vi "parser.vi"(11 "input string":string) -> ()   [LabVIEW 2014]
panel:
  out "element":i32
  out "errorstate":string
  out "error":bool
  in  "Listbox":i32(listbox)
  out "Enum":enum16{"%g", "bias", "current", "frame"}(ring)
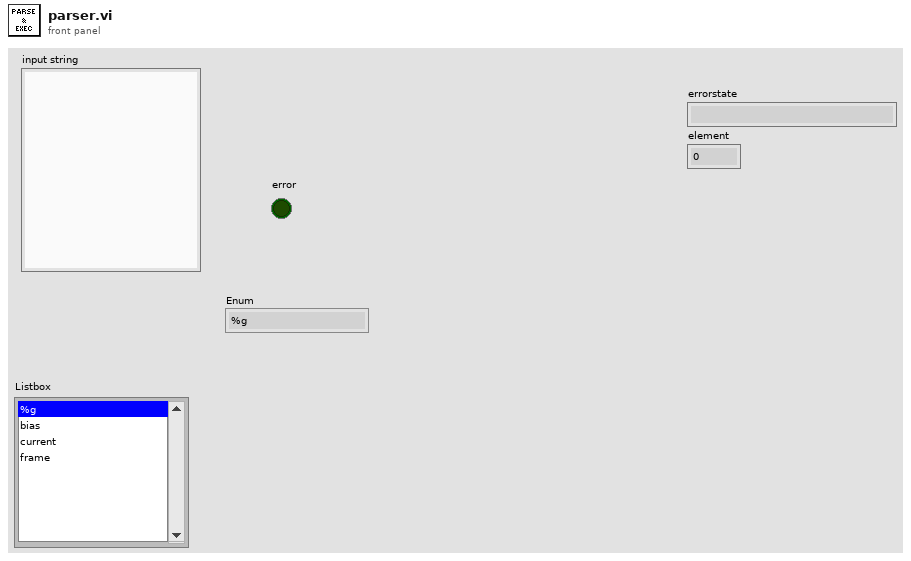
[diagram p1: front panel]
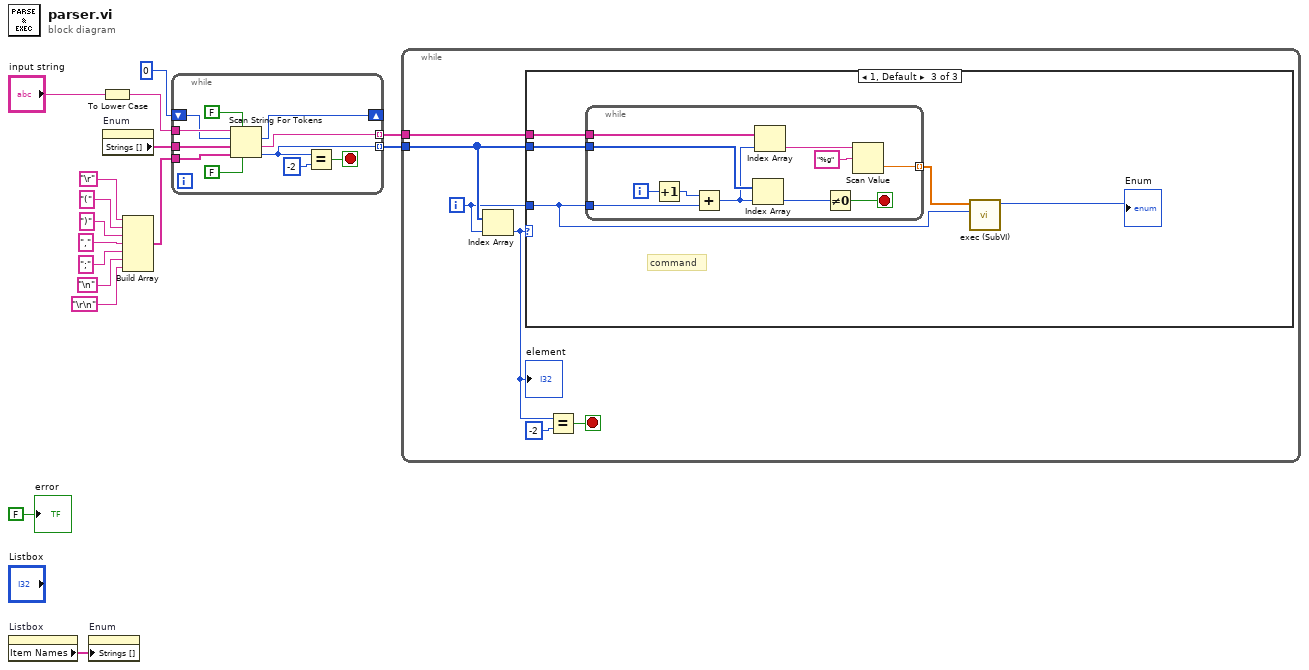
[diagram p0: block diagram]
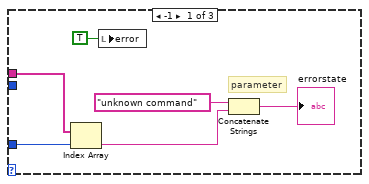
[diagram p2: hidden frame]
diagram:
  n1 = property on="Listbox" class="LstBox (strict)"() -> ("Item Names"=w4:string[])  [unwired: 2 in, 2 out]
  n2 = property on="Enum" class="Enum (strict)"("Strings []"=w4) -> ()  [unwired: 2 in, 2 out]
  n3 = To Lower Case(string="input string") -> (all lower case string=w10:string)
  n4 = property on="Enum" class="Enum (strict)"() -> ("Strings []"=w5:string[])  [unwired: 2 in, 2 out]
  n5 = Build Array("\r", "(" ("element"), ")" ("element"), "," ("element"), ";" ("element"), "\n", "\r\n") -> (w15:string[])
  n6 = while {
    tunnel: w15 -> [w27]
    tunnel: [w25] -> w6 mode=indexing
    tunnel: w5 -> [w18]
    tunnel: w10 -> [w24]
    shift-right: [w20] -> _
    shift-left: 0 ("y") -> [w21]
    tunnel: [w19] -> w7 mode=indexing
    stop <- w23 stop-if-true
    n7 = Scan String For Tokens(4:FALSE ("use cached delim/oper data? (F)"), 5:FALSE ("allow empty tokens? (F)"), 6:w27, 7:w18, 8:w21, 9:w24) -> (0:w19:i32, 1:w25:string, 2:w20:i32)  [unwired: 1 out]
    n8 = Equal?(x=w19, y=-2) -> (x = y?=w23:bool)
  }
  n9 = while {
    tunnel: w7 -> [w31]
    tunnel: w6 -> [w29]
    i -> [w30]
    stop <- w32 stop-if-true
    n10 = Index Array(array=w31, index=w30) -> (element=w28:i32)
    "element" <- w28
    n11 = case shown="1, Default" w28 {
      tunnel: w31 -> [_ _ w44]
      tunnel: w30 -> [w37 _ w42]
      tunnel: w29 -> [w38 _ w43]
      frame -1 {
        # "parameter"
        n12 = Index Array(array=w38, index=w37) -> (element=w36:string)
        n13 = local write "error"(TRUE ("error")) -> ()
        n14 = Concatenate Strings("unknown command" ("string"), w36) -> (→"errorstate":string)
      }
      frame -2, 0 {
      }
      frame 1, Default {
        # "command"
        n15 = while {
          tunnel: w44 -> [w55]
          tunnel: w42 -> [w53]
          tunnel: w43 -> [w49]
          tunnel: [w45] -> w41 mode=indexing
          i -> [w52]
          stop <- w54 stop-if-true
          n16 = Increment(x=w52) -> (x+1=w51:i32)
          n17 = Add(x=w51, y=w53) -> (x+y=w48:i32)
          n18 = Index Array(array=w55, index=w48) -> (element=w50:i32)
          n19 = Index Array(array=w49, index=w48) -> (element=w47:string)
          n20 = Not Equal To 0?(x=w50) -> (x != 0?=w54:bool)
          n21 = Scan Value(string=w47, format string="%g") -> (value=w45:dbl)  [unwired: 1 in, 1 out]
        }
        n22 = call "exec (SubVI).vi"("Numeric"=w42, "Array"=w41) -> ("Enum"=→"Enum":enum16{"%g", "bias", "current", "frame"})  [unwired: 9 in]
      }
    }
    n23 = Equal?(x=w28, y=-2) -> (x = y?=w32:bool)
  }
  "error" <- FALSE ("error")
